vi "MotorUI.vi"() -> ()   [LabVIEW 2011]
uses:
  MotorPosType.ctl
  Typedefs/XYf.ctl
  MotorStateType.ctl
  Typedefs/CmdEnum_MotorIn.ctl
  MotorAxisEnum.ctl
  MotorCmd_MoveToLimit.ctl
  GlobalVariables.vi
panel:
  in  "Save config":bool
  in  "Piezo XY":T1
  out "Piezo Y":sgl
  out "Piezo X":sgl
  out "Focal depth (um):":sgl
  out "Rotation (turns):":sgl
  out "Position: (mm)":sgl
  out "Motor update lag counter":i32
  in  "Rotation speed\n(turns/s)":sgl=1.0
  in  "Magnet offset":sgl
  in  "Piezo step pageup/down":sgl=2.0
  in  "Magnet home":bool
  in  "Reset magnet zero pos":bool
  out "Offset":T2
  in  "MotorState (initial value)":T3
  in  "Step size of up/down buttons":sgl=3.0
  in  "Motors Initialized?":bool
  out "motor cmd queue len":i32
  out "Current Position":T2
  in  "Piezo position":sgl
  in  "Magnet position [mm]":sgl
  in  "Rotation [turns]":sgl
  in  "Move magnet up":bool
  in  "Move magnet down":bool
  in  "Magnet rotation: Alternate 0/10":bool
  in  "Piezo stage down":bool
  in  "Piezo stage up":bool
  in  "Piezo step:":sgl=5.0
  # "Magnet Z"
  # "Focal depth"
  # "Magnet Rotation"
  # "Piezo XY"
  # "Magnet position:\nThe shown 'magnet position' cannot go below zero, so you can use the offset to set a lower magnet limit (in order to protect your flowcell)"
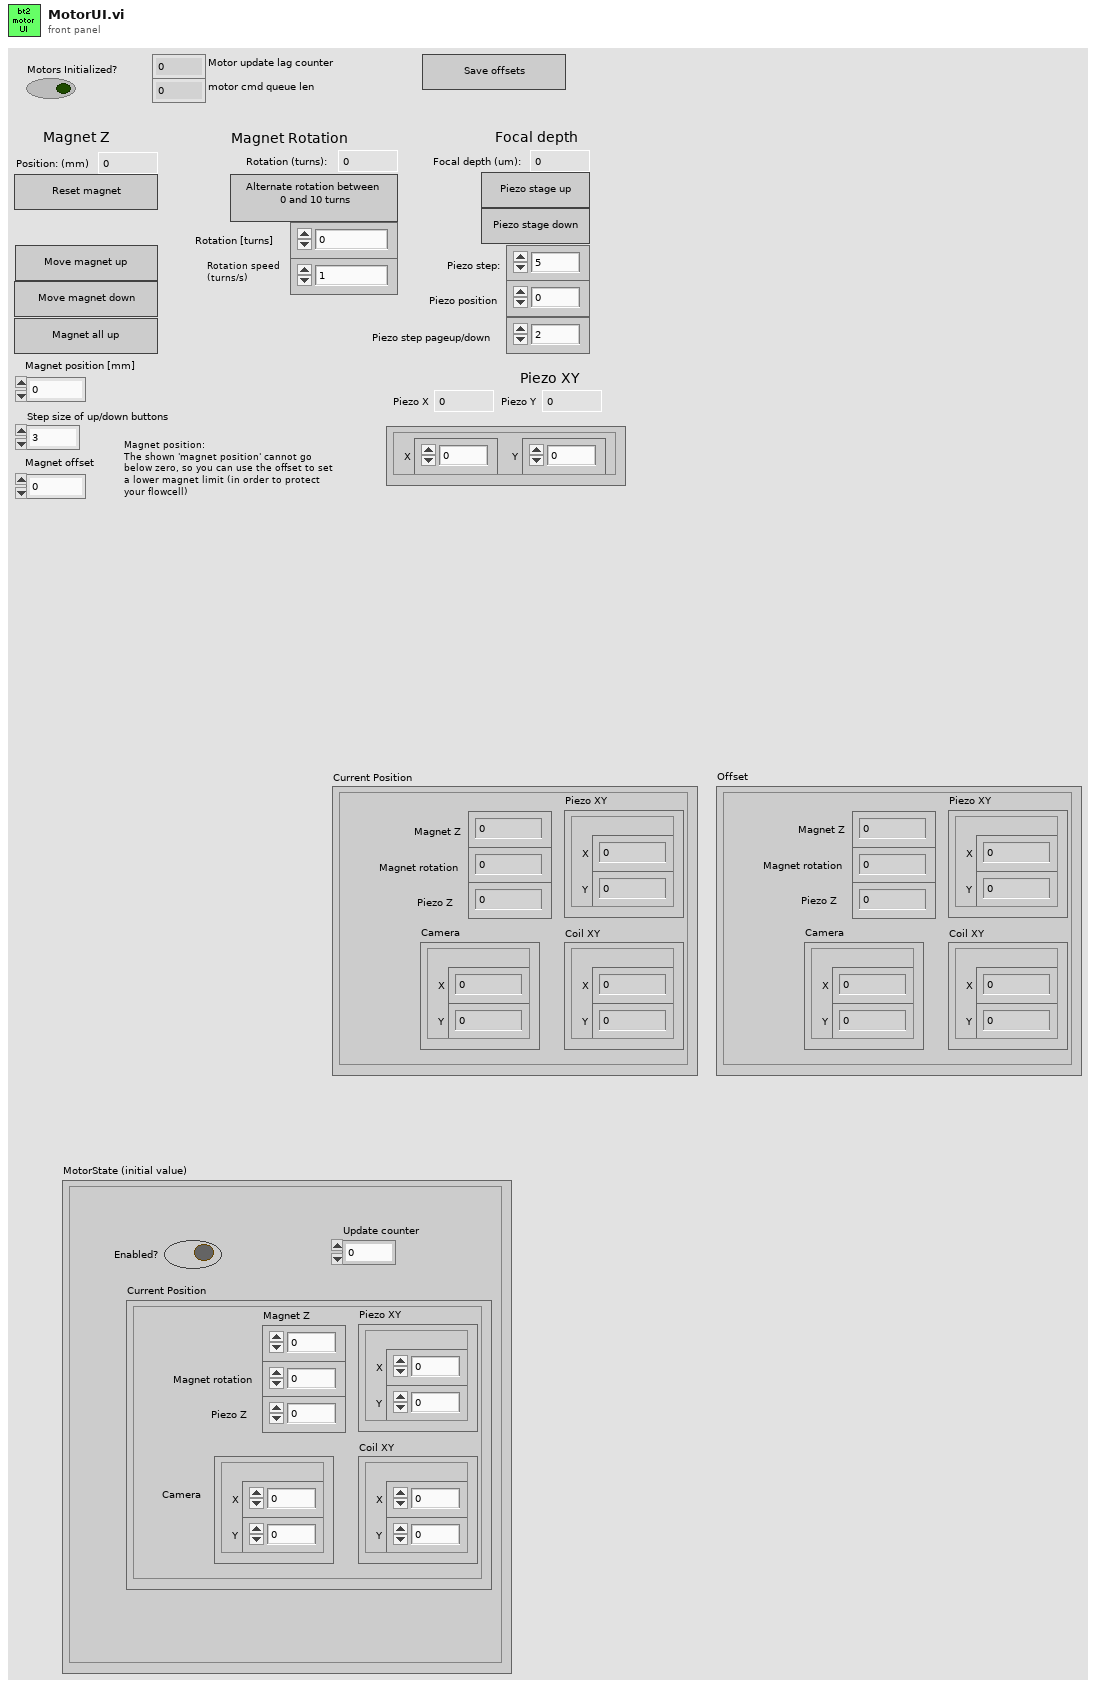
[diagram p1: front panel]
types:
  T1 = typedef "XYf.ctl" = cluster{"X":sgl, "Y":sgl}
  T2 = typedef "MotorPosType.ctl" = cluster{"Magnet Z":dbl, "Magnet rotation":dbl, "Camera":T1, "Piezo XY":T1, "Piezo Z":dbl, "Coil XY":T1}
  T3 = typedef "MotorStateType.ctl" = cluster{"Enabled?":bool, "Current Position":T2, "Update counter":i32}
  T4 = typedef "MotorConfigType.ctl" = cluster{"Offset":T2, "Maximum pos":T2, "Min limited?":T5, "Max limited?":T5, "Has velocity support":T5, "Default velocity":T2}
  T5 = typedef "MotorPosFlagsType.ctl" = cluster{"Magnet Z":bool, "Magnet rotation":bool, "Camera":cluster{"X":bool, "Y":bool}, "Piezo XY":cluster{"X":bool, "Y":bool}, "Piezo Z":bool, "Coil XY":cluster{"X":bool, "Y":bool}}
  T6 = typedef "MotorAxisEnum.ctl" = enum16{"no axis", "magrot", "magpos", "px", "py", "pz", "camx", "camy"}
  T7 = typedef "CmdEnum_MotorIn.ctl" = enum32{"Init", "Close", "SetPosition", "UpdatePositions", "MoveToLimit"}
  T8 = typedef "MotorCmd_MoveToLimit.ctl" = cluster{"Motor Axis":T6, "Limit switch":enum16{"Positive", "Negative"}}
  T9 = typedef "eventvkey.ctl" = enum16{"ASCII", "Enter", "Return", "Shift", "Ctrl", "Alt", "Cmd", "Opt", "Caps", "NumLock", "Clear", "Break", "Up", "Down", "Left", "Right", "Insert", "Delete", "Home", "End", "PageUp", "PageDown", "Escape", "Help", "Pause", "ScrollLock", "F1", "F2", "F3", "F4", "F5", "F6", "F7", "F8", "F9", "F10", "F11", "F12", "F13", "F14", "F15", "F16", "F17", "F18", "F19", "F20", "F21", "F22", "F23", "F24", "Play", "VolumeUp", "VolumeDown", "Mute", "Two Byte Char"}
  T10 = typedef "QueueListType.ctl" = cluster{"Motor In":refnum<queue>, "User Interface Image View":refnum<queue>, "User Interface Camera Control":refnum<queue>, "User Interface Event Notifier":refnum<notifier>, "Initialized?":bool}
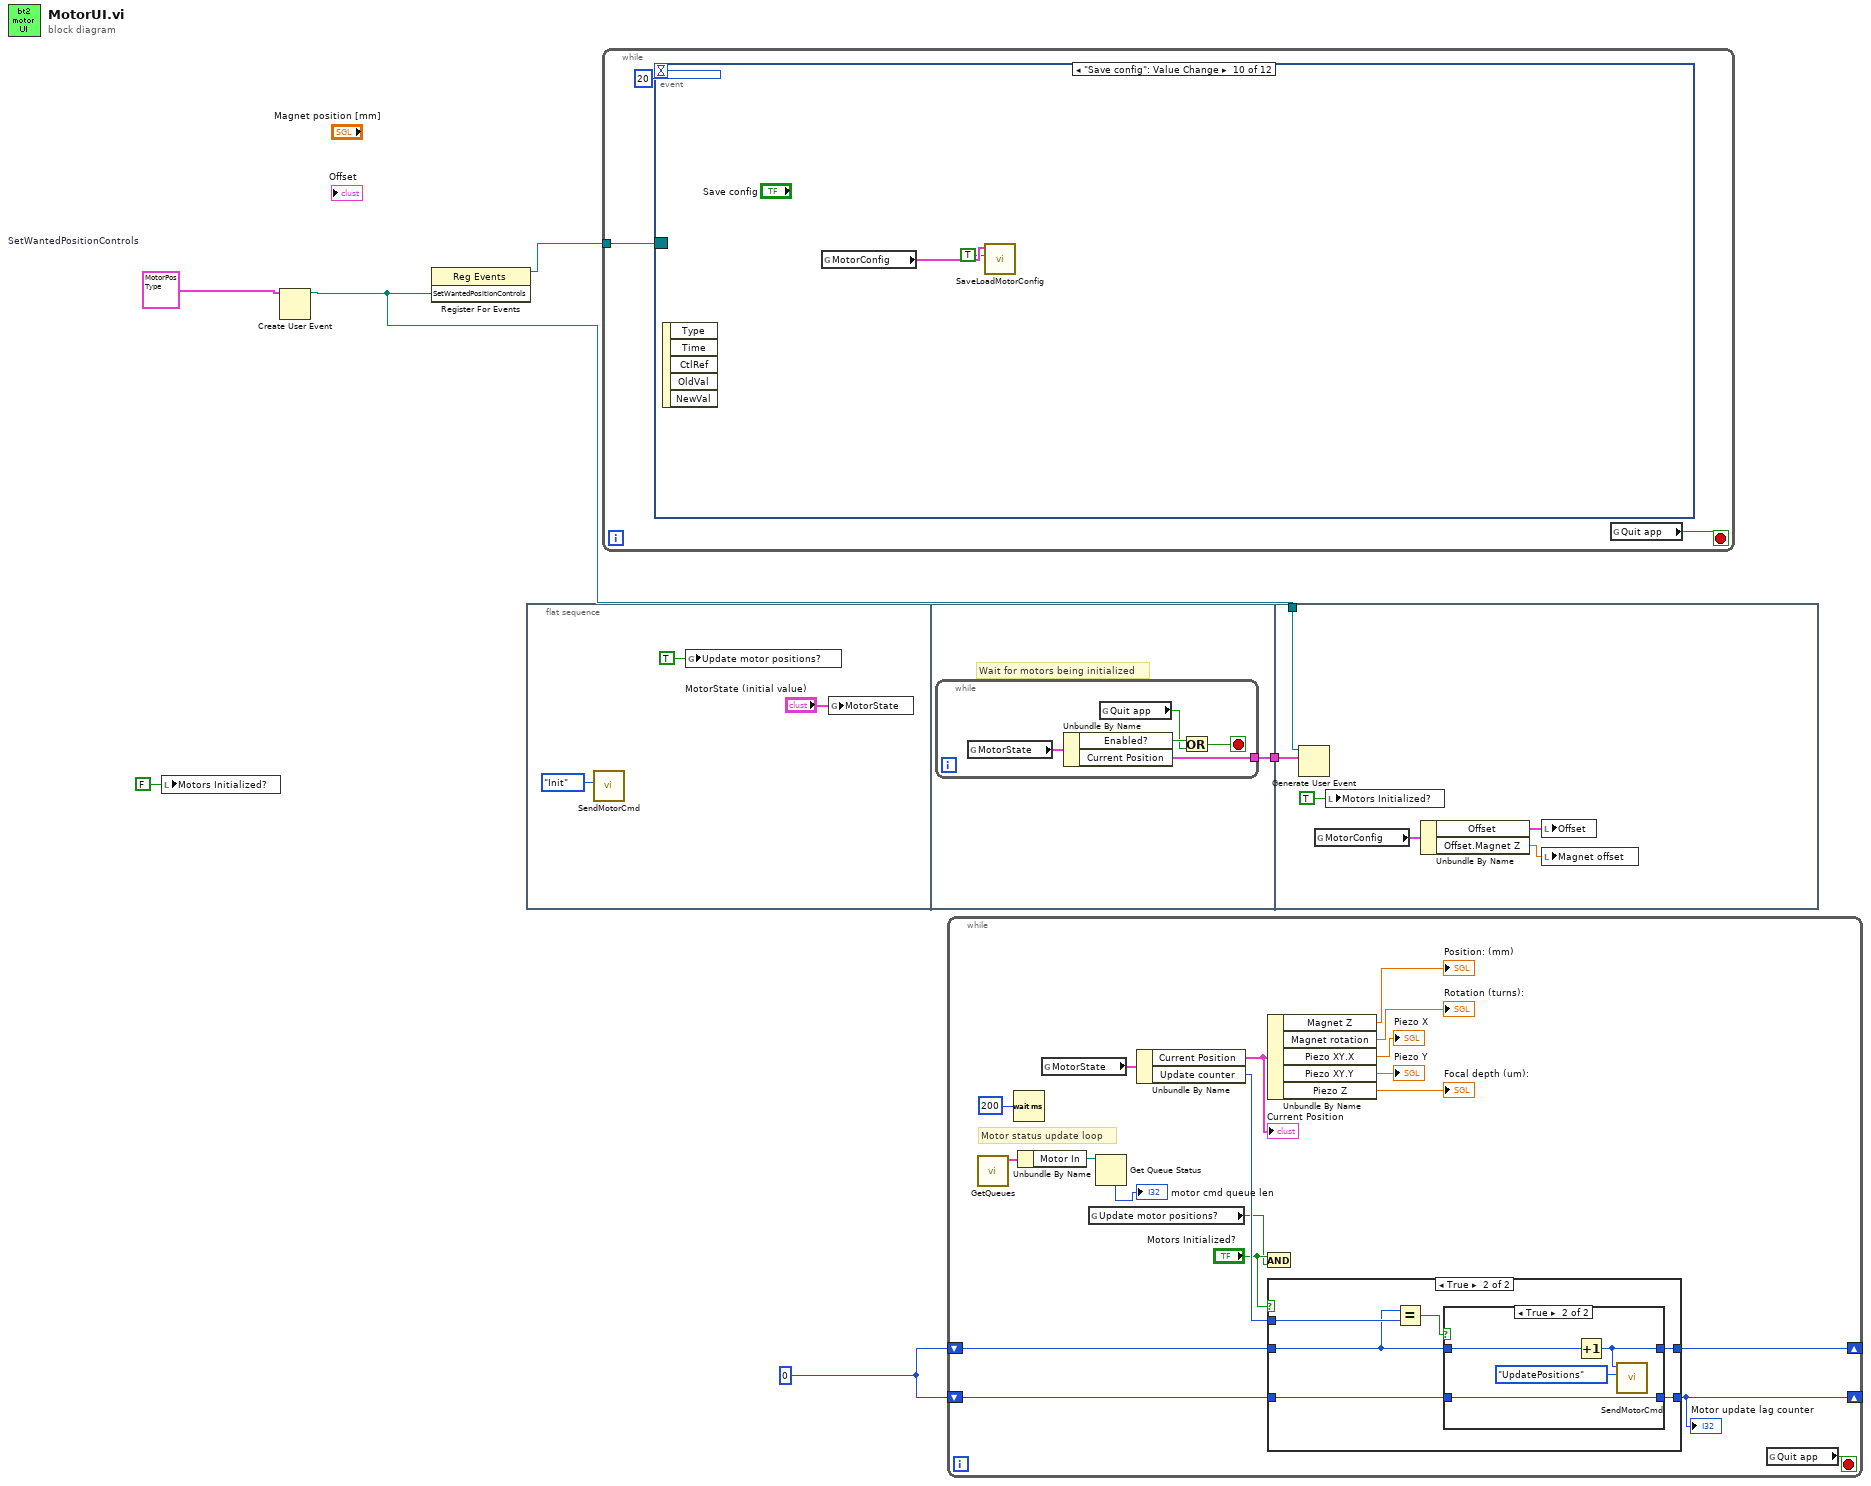
[diagram p0: block diagram]
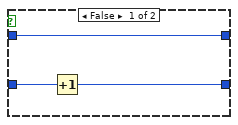
[diagram p3: hidden frame]
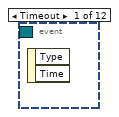
[diagram p4: hidden frame]
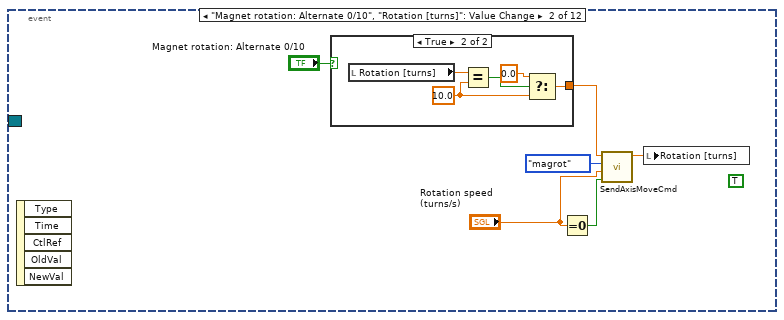
[diagram p5: hidden frame]
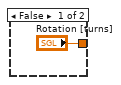
[diagram p6: hidden frame]
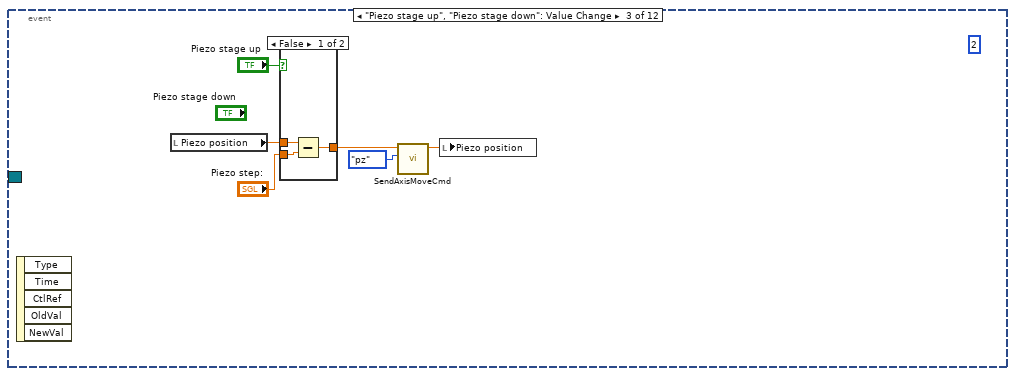
[diagram p7: hidden frame]
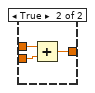
[diagram p8: hidden frame]
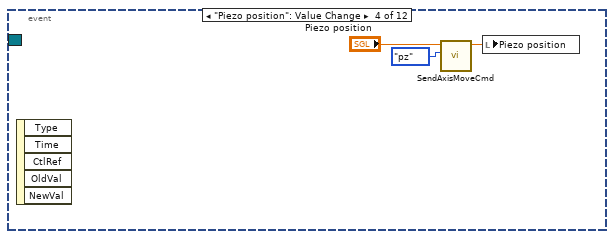
[diagram p9: hidden frame]
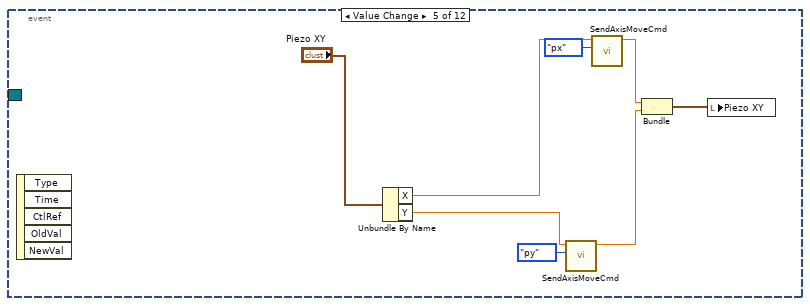
[diagram p10: hidden frame]
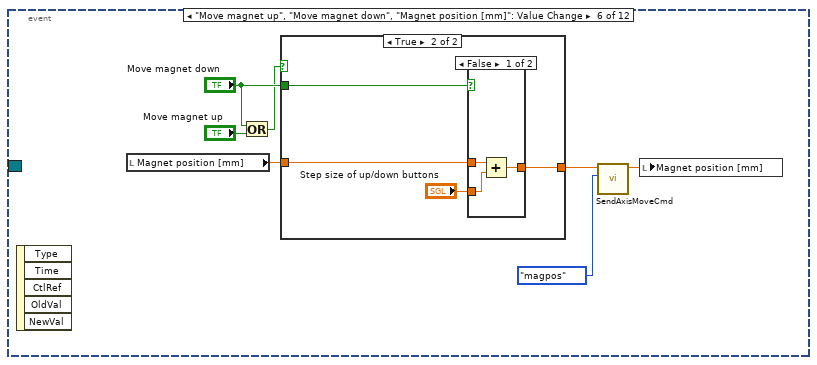
[diagram p11: hidden frame]
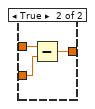
[diagram p13: hidden frame]
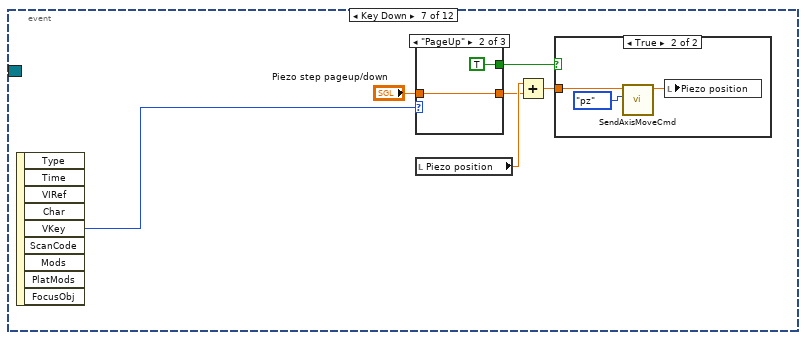
[diagram p14: hidden frame]
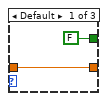
[diagram p16: hidden frame]
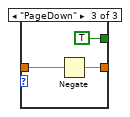
[diagram p17: hidden frame]
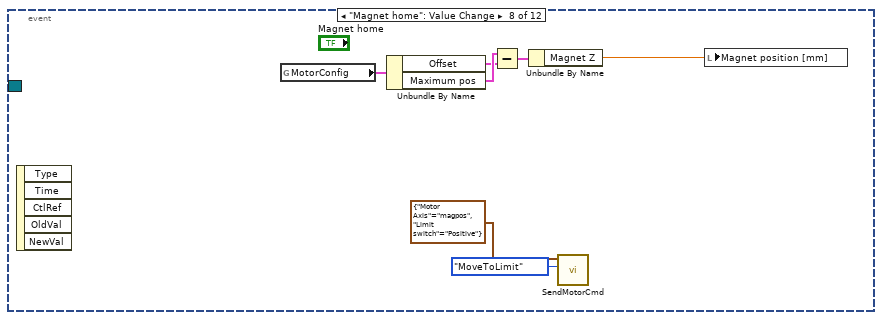
[diagram p18: hidden frame]
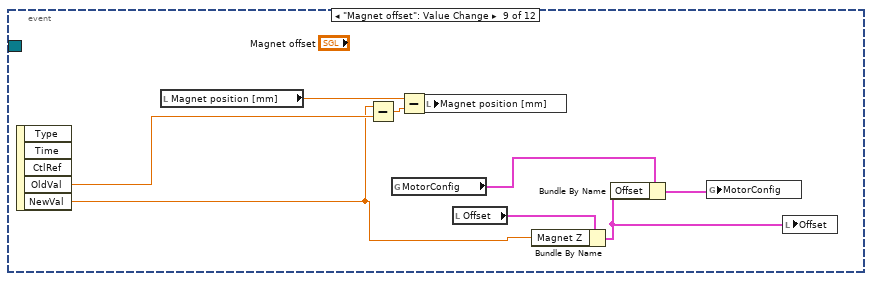
[diagram p19: hidden frame]
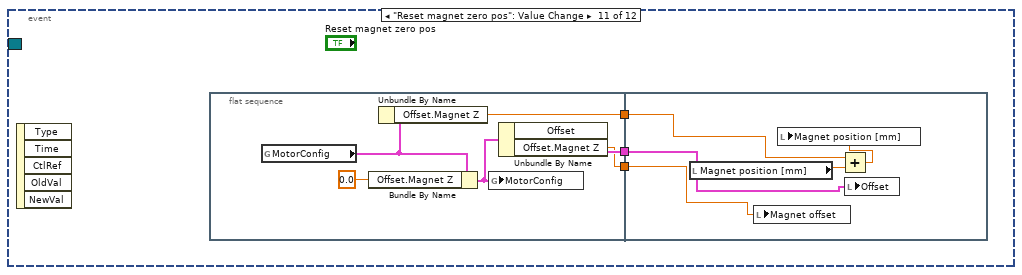
[diagram p20: hidden frame]
diagram:
  w4 = 0 ("Update counter")
  w5 = T2 {"Magnet Z"=0.0, "Magnet rotation"=0.0, "Camera"={"X"=0.0, "Y"=0.0}, "Piezo XY"={"X"=0.0, "Y"=0.0}, "Piezo Z"=0.0, "Coil XY"={"X"=0.0, "Y"=0.0}}  # SetWantedPositionControls
  n1 = local write "Motors Initialized?"(FALSE ("Motor Initialized?")) -> ()
  n2 = Create User Event(user event datatype=w5) -> (user event=w1:refnum<user-event>)  [unwired: 1 in, 1 out]
  n3 = register-events(w1) -> (reference out=w3:refnum<event-registration>)  [unwired: 2 in, 1 out]
  n4 = flat-sequence {
    tunnel: [w10] -> w2
    tunnel: w1 -> [w20]
    tunnel: w2 -> [w19]
    frame #0 {
      n5 = call "SendMotorCmd.vi"("Command Type"=enum16{"Init", "Close", "SetPosition"}."Init") -> ()  [unwired: 11 in]
      n6 = global write "GlobalVariables.vi" "Update motor positions?"(TRUE ("Update motor positions?")) -> ()
      n7 = global write "GlobalVariables.vi" "MotorState"("MotorState (initial value)") -> ()
    }
    frame #1 {
      # "Wait for motors being initialized"
      n8 = while {
        tunnel: [w14] -> w10
        stop <- w11 stop-if-true
        n9 = global read "GlobalVariables.vi" "MotorState"() -> (w15:T3)
        n10 = Unbundle By Name(w15) -> ("Enabled?"=w13:bool, "Current Position"=w14:T2)
        n11 = global read "GlobalVariables.vi" "Quit app"() -> (w12:bool)
        n12 = Or(x=w13, y=w12) -> (x .or. y?=w11:bool)
      }
    }
    frame #2 {
      n13 = Generate User Event(user event=w20, event data cluster=w19) -> ()  [unwired: 1 in, 2 out]
      n14 = global read "GlobalVariables.vi" "MotorConfig"() -> (w18:T4)
      n15 = local write "Motors Initialized?"(TRUE ("Motor Initialized?")) -> ()
      n16 = Unbundle By Name(w18) -> ("Offset"=w16:T2, "Offset.Magnet Z"=w17:dbl)
      n17 = local write "Offset"(w16) -> ()
      n18 = local write "Magnet offset"(w17) -> ()
    }
  }
  n19 = while {
    tunnel: w3 -> [w22]
    stop <- w23 stop-if-true
    n20 = event shown="[9] \"Save config\": Value Change" {
      selector: w22 -> [_ _ _ _ _ _ _ _ _ _ _ _]
      dyn-events: _ -> [_ _ _ _ _ _ _ _ _ _ _ _]
      timeout: 20 -> [_ _ _ _ _ _ _ _ _ _ _ _]
      event Timeout {
        n21 = event-data() -> ()  [unwired: 1 in, 2 out]
      }
      event "Magnet rotation: Alternate 0/10", "Rotation [turns]": Value Change {
        (unwired) TRUE ("Move flags.Magnet rotation")
        n22 = event-data() -> ()  [unwired: 1 in, 5 out]
        n23 = case shown="True" "Magnet rotation: Alternate 0/10" {
          tunnel: ["Rotation [turns]" w32] -> w28
          frame False {
          }
          frame True {
            w33 = sgl 10.0 ("y")
            n24 = local read "Rotation [turns]"() -> (w36:sgl)
            n25 = Equal?(x=w36, y=w33) -> (x = y?=w35:bool)
            n26 = Select(t=0.0, s=w35, f=w33) -> (s? t:f=w32:dbl)
          }
        }
        n27 = Equal To 0?(x="Rotation speed\n(turns/s)") -> (x = 0?=w25:bool)
        n28 = call "SendAxisMoveCmd.vi"("Instant? (T)"=w25, "Speed"="Rotation speed\n(turns/s)", "axis"=MotorAxisEnum."magrot", "Position"=w28) -> ("Limited pos"=w29:dbl)  [unwired: 7 in]
        n29 = local write "Rotation [turns]"(w29) -> ()
      }
      event "Piezo stage up", "Piezo stage down": Value Change {
        (unwired) 2 ("axis index")
        n30 = event-data() -> ()  [unwired: 1 in, 5 out]
        n31 = local read "Piezo position"() -> (w40:sgl)
        n32 = case shown="False" "Piezo stage up" {
          tunnel: w40 -> [w45 w48]
          tunnel: "Piezo step:" -> [w44 w47]
          tunnel: [w43 w46] -> w38
          frame False {
            n33 = Subtract(x=w45, y=w44) -> (x-y=w43:sgl)
          }
          frame True {
            n34 = Add(x=w48, y=w47) -> (x+y=w46:sgl)
          }
        }
        n35 = call "SendAxisMoveCmd.vi"("axis"=MotorAxisEnum."pz", "Position"=w38) -> ("Limited pos"=w39:dbl)  [unwired: 9 in]
        n36 = local write "Piezo position"(w39) -> ()
      }
      event "Piezo position": Value Change {
        n37 = event-data() -> ()  [unwired: 1 in, 5 out]
        n38 = call "SendAxisMoveCmd.vi"("axis"=MotorAxisEnum."pz", "Position"="Piezo position") -> ("Limited pos"=w49:dbl)  [unwired: 9 in]
        n39 = local write "Piezo position"(w49) -> ()
      }
      event Value Change {
        n40 = event-data() -> ()  [unwired: 1 in, 5 out]
        n41 = Unbundle By Name("Piezo XY") -> ("X"=w58:sgl, "Y"=w57:sgl)
        n42 = call "SendAxisMoveCmd.vi"("axis"=MotorAxisEnum."py", "Position"=w57) -> ("Limited pos"=w53:dbl)  [unwired: 9 in]
        n43 = call "SendAxisMoveCmd.vi"("axis"=MotorAxisEnum."px", "Position"=w58) -> ("Limited pos"=w54:dbl)  [unwired: 9 in]
        n44 = Bundle("Limited pos"=w54, "Limited pos"=w53) -> (w52:cluster{"Limited pos":dbl, "Limited pos":dbl})  [unwired: 1 in]
        n45 = local write "Piezo XY"(w52) -> ()
      }
      event "Move magnet up", "Move magnet down", "Magnet position [mm]": Value Change {
        n46 = event-data() -> ()  [unwired: 1 in, 5 out]
        n47 = local read "Magnet position [mm]"() -> (w63:sgl)
        n48 = Or(x="Move magnet down", y="Move magnet up") -> (x .or. y?=w64:bool)
        n49 = case shown="True" w64 {
          tunnel: w63 -> [w67 w71]
          tunnel: "Move magnet down" -> [_ w69]
          tunnel: [w67 w68] -> w61
          frame False {
          }
          frame True {
            n50 = case shown="False" w69 {
              tunnel: w71 -> [w74 w77]
              tunnel: "Step size of up/down buttons" -> [w73 w76]
              tunnel: [w72 w75] -> w68
              frame False {
                n51 = Add(x=w74, y=w73) -> (x+y=w72:sgl)
              }
              frame True {
                n52 = Subtract(x=w77, y=w76) -> (x-y=w75:sgl)
              }
            }
          }
        }
        n53 = call "SendAxisMoveCmd.vi"("axis"=MotorAxisEnum."magpos", "Position"=w61) -> ("Limited pos"=w60:dbl)  [unwired: 9 in]
        n54 = local write "Magnet position [mm]"(w60) -> ()
      }
      event Key Down {
        n55 = event-data() -> ("VKey"=w83:T9)  [unwired: 1 in, 8 out]
        n56 = case shown="\"PageUp\"" w83 {
          tunnel: [FALSE TRUE TRUE] -> w82
          tunnel: "Piezo step pageup/down" -> [w87 w89 w92]
          tunnel: [w87 w89 w91] -> w79
          frame Default {
          }
          frame "PageUp" {
          }
          frame "PageDown" {
            n57 = Negate(x=w92) -> (-x=w91:sgl)
          }
        }
        n58 = local read "Piezo position"() -> (w80:sgl)
        n59 = Add(x=w80, y=w79) -> (x+y=w78:sgl)
        n60 = case shown="True" w82 {
          tunnel: w78 -> [_ w85]
          frame False {
          }
          frame True {
            n61 = call "SendAxisMoveCmd.vi"("axis"=MotorAxisEnum."pz", "Position"=w85) -> ("Limited pos"=w84:dbl)  [unwired: 9 in]
            n62 = local write "Piezo position"(w84) -> ()
          }
        }
      }
      event "Magnet home": Value Change {
        n63 = event-data() -> ()  [unwired: 1 in, 5 out]
        n64 = global read "GlobalVariables.vi" "MotorConfig"() -> (w100:T4)
        n65 = Unbundle By Name(w100) -> ("Offset"=w98:T2, "Maximum pos"=w99:T2)
        n66 = Subtract(x=w99, y=w98) -> (x-y=w97:T2)
        n67 = Unbundle By Name(w97) -> ("Magnet Z"=w94:dbl)
        n68 = call "SendMotorCmd.vi"("Command Type"=CmdEnum_MotorIn."MoveToLimit", "Command Data"=T8 {"Motor Axis"=enum."magpos", "Limit switch"=enum."Positive"} ("MotorCmd_MoveToLimit")) -> ()  [unwired: 10 in]
        n69 = local write "Magnet position [mm]"(w94) -> ()
      }
      event "Magnet offset": Value Change {
        n70 = event-data() -> ("OldVal"=w109:sgl, "NewVal"=w102:sgl)  [unwired: 1 in, 3 out]
        n71 = local read "Magnet position [mm]"() -> (w108:sgl)
        n72 = Subtract(x=w102, y=w109) -> (x-y=w107:sgl)
        n73 = global read "GlobalVariables.vi" "MotorConfig"() -> (w105:T4)
        n74 = Subtract(x=w108, y=w107) -> (x-y=w106:sgl)
        n75 = local write "Magnet position [mm]"(w106) -> ()
        n76 = local read "Offset"() -> (w103:T2)
        n77 = Bundle By Name(cluster=w103, "Magnet Z"=w102) -> (w101:T2)
        n78 = Bundle By Name(cluster=w105, "Offset"=w101) -> (w104:T4)
        n79 = global write "GlobalVariables.vi" "MotorConfig"(w104) -> ()
        n80 = local write "Offset"(w101) -> ()
      }
      event "Save config": Value Change {
        n81 = event-data() -> ()  [unwired: 1 in, 5 out]
        n82 = global read "GlobalVariables.vi" "MotorConfig"() -> (w111:T4)
        n83 = call "SaveLoadMotorConfig.vi"("Save? (F)"=TRUE ("Save?"), "MotorConfig(in)"=w111) -> ()  [unwired: 7 in, 3 out]
      }
      event "Reset magnet zero pos": Value Change {
        n84 = event-data() -> ()  [unwired: 1 in, 5 out]
        n85 = flat-sequence {
          tunnel: [w118] -> w114
          tunnel: [w116] -> w113
          tunnel: [w115] -> w112
          tunnel: w114 -> [w124]
          tunnel: w113 -> [w122]
          tunnel: w112 -> [w121]
          frame #0 {
            n86 = global read "GlobalVariables.vi" "MotorConfig"() -> (w119:T4)
            n87 = Bundle By Name(cluster=w119, "Offset.Magnet Z"=0.0) -> (w117:T4)
            n88 = Unbundle By Name(w119) -> ("Offset.Magnet Z"=w118:dbl)
            n89 = global write "GlobalVariables.vi" "MotorConfig"(w117) -> ()
            n90 = Unbundle By Name(w117) -> ("Offset"=w116:T2, "Offset.Magnet Z"=w115:dbl)
          }
          frame #1 {
            n91 = local read "Magnet position [mm]"() -> (w125:sgl)
            n92 = local write "Magnet offset"(w121) -> ()
            n93 = Add(x=w124, y=w125) -> (x+y=w123:dbl)
            n94 = local write "Magnet position [mm]"(w123) -> ()
            n95 = local write "Offset"(w122) -> ()
          }
        }
      }
      event User Event {
        n96 = event-data() -> ("Magnet Z"=w129:dbl, "Magnet rotation"=w128:dbl, "Piezo XY"=w126:T1, "Piezo Z"=w127:dbl)  [unwired: 1 in, 4 out]
        n97 = local write "Piezo position"(w127) -> ()
        n98 = local write "Magnet position [mm]"(w129) -> ()
        n99 = local write "Rotation [turns]"(w128) -> ()
        n100 = local write "Piezo XY"(w126) -> ()
      }
    }
    n101 = global read "GlobalVariables.vi" "Quit app"() -> (w23:bool)
  }
  n102 = while {
    shift-right: [w140] -> _
    shift-left: w4 -> [w141]
    shift-right: [w138] -> _
    shift-left: w4 -> [w139]
    stop <- w147 stop-if-true
    # "Motor status update loop"
    n103 = call "GetQueues.vi"() -> ("Queue List"=w145:T10)  [unwired: 10 in, 1 out]
    n104 = Wait (ms)(milliseconds to wait=u32 200) -> ()  [unwired: 1 out]
    n105 = Unbundle By Name(w145) -> ("Motor In"=w144:refnum<queue>)
    n106 = global read "GlobalVariables.vi" "MotorState"() -> (w146:T3)
    n107 = global read "GlobalVariables.vi" "Update motor positions?"() -> (w136:bool)
    n108 = Get Queue Status(queue=w144) -> (# elements in queue=→"motor cmd queue len":i32)  [unwired: 2 in, 7 out]
    n109 = Unbundle By Name(w146) -> ("Current Position"=w135:T2, "Update counter"=w142:i32)
    "Current Position" <- w135
    n110 = And(x="Motors Initialized?", y=w136) -> ()  [unwired: 1 out]
    n111 = Unbundle By Name(w135) -> ("Magnet Z"=→"Position: (mm)":dbl, "Magnet rotation"=→"Rotation (turns):":dbl, "Piezo XY.X"=→"Piezo X":sgl, "Piezo XY.Y"=→"Piezo Y":sgl, "Piezo Z"=→"Focal depth (um):":dbl)
    n112 = case shown="True" "Motors Initialized?" {
      tunnel: w142 -> [_ w156]
      tunnel: w141 -> [w150 w152]
      tunnel: [w150 w151] -> w140
      tunnel: w139 -> [w149 w154]
      tunnel: [w149 w153] -> w138
      frame False {
      }
      frame True {
        n113 = Equal?(x=w152, y=w156) -> (x = y?=w155:bool)
        n114 = case shown="True" w155 {
          tunnel: w152 -> [w157 w161]
          tunnel: w154 -> [w159 w162]
          tunnel: [w158 w162] -> w153
          tunnel: [w157 w160] -> w151
          frame False {
            n115 = Increment(x=w159) -> (x+1=w158:i32)
          }
          frame True {
            n116 = Increment(x=w161) -> (x+1=w160:i32)
            n117 = call "SendMotorCmd.vi"("Command Type"=CmdEnum_MotorIn."UpdatePositions", "Command Data"=w160) -> ()  [unwired: 10 in]
          }
        }
      }
    }
    "Motor update lag counter" <- w138
    n118 = global read "GlobalVariables.vi" "Quit app"() -> (w147:bool)
  }
